vi "misurazione_distanza(subVI).vi"(8 "error in (no error)":errorcluster, 9 "punto 1":i32=1, 10 "punto 0":i32, 11 "particle reports (real-world)":T1(array[cluster])) -> (0 "error out":errorcluster, 3 "Distances":sgl[](array[numeric]) format="%.4f")   [LabVIEW 2020]
uses:
  <vilib>/vision/NI_Vision_Development_Module.lvlib
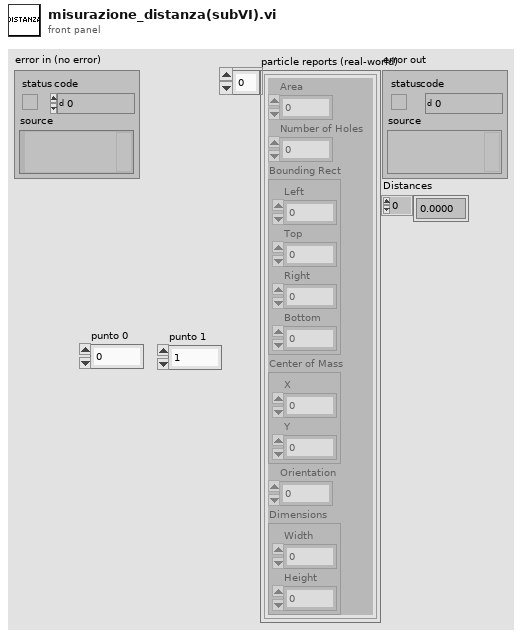
[diagram p1: front panel]
types:
  T1 = cluster{"Area":dbl, "Number of Holes":dbl, "Bounding Rect":cluster{"Left":dbl, "Top":dbl, "Right":dbl, "Bottom":dbl}, "Center of Mass":cluster{"X":dbl, "Y":dbl}, "Orientation":dbl, "Dimensions":cluster{"Width":dbl, "Height":dbl}}[]
  T2 = cluster{"Area":dbl, "Number of Holes":dbl, "Bounding Rect":cluster{"Left":dbl, "Top":dbl, "Right":dbl, "Bottom":dbl}, "Center of Mass":cluster{"X":dbl, "Y":dbl}, "Orientation":dbl, "Dimensions":cluster{"Width":dbl, "Height":dbl}}
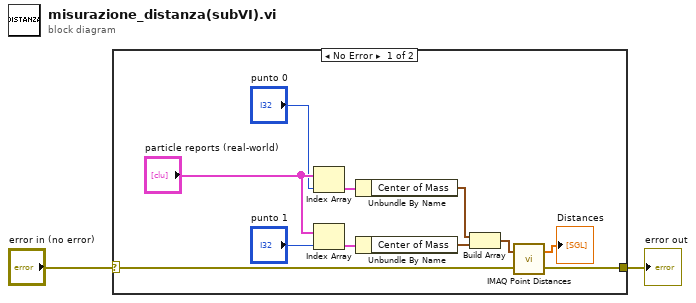
[diagram p0: block diagram]
diagram:
  n1 = case shown="No Error" "error in (no error)" {
    selector: "error in (no error)" -> [w7 w14]
    tunnel: [w8 w14] -> w2
    frame No Error {
      n2 = Index Array(array="particle reports (real-world)", index="punto 0") -> (element=w11:T2)
      n3 = Index Array(array="particle reports (real-world)", index="punto 1") -> (element=w10:T2)
      n4 = Unbundle By Name(w11) -> ("Center of Mass"=w13:cluster{"X":dbl, "Y":dbl})
      n5 = Unbundle By Name(w10) -> ("Center of Mass"=w12:cluster{"X":dbl, "Y":dbl})
      n6 = Build Array(w13, w12) -> (w9:cluster{"X":dbl, "Y":dbl}[])
      n7 = call "IMAQ Point Distances"("Points"=w9, "error in (no error)"=w7) -> ("Distances"=→"Distances":sgl[], "error out"=w8:errorcluster)  [unwired: 3 in]
    }
    frame Error {
    }
  }
  "error out" <- w2
